vi "Delete Alarm archive and Create Header for new one Alarm archive.vi"(8 "error in":errorcluster) -> (0 "error out":errorcluster)   [LabVIEW 2023]
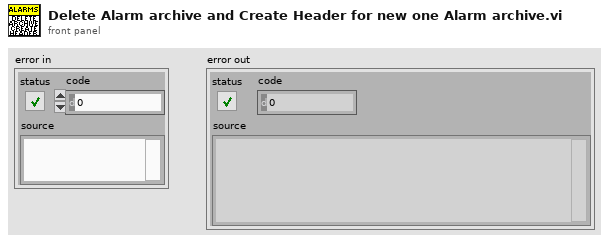
[diagram p1: front panel]
types:
  T1 = enum16{"open", "replace", "create", "open or create", "replace or create", "replace or create with confirmation"}
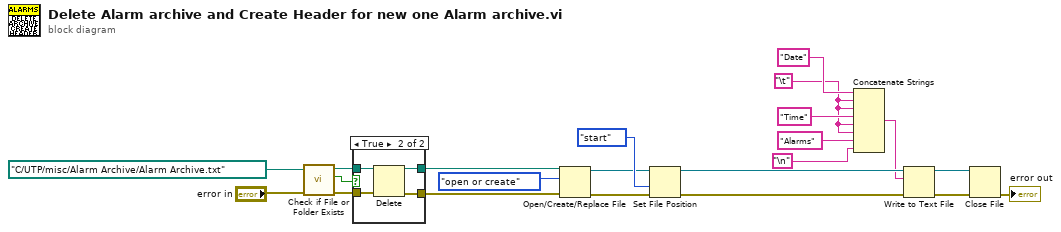
[diagram p0: block diagram]
diagram:
  w12 = "\t"
  n1 = call <vilib>:"Check if File or Folder Exists.vi"("error in (no error)"="error in", "path"=path "C:/UTP/misc/Alarm Archive/Alarm Archive.txt" ("file path (use dialog)")) -> ("error out"=w1:errorcluster, "file or folder exists?"=w2:bool, "dup path"=w3:path)  [unwired: 7 in]
  n2 = case shown="True" w2 {
    tunnel: [w24 w28] -> w7
    tunnel: [w23 w27] -> w6
    tunnel: w3 -> [w24 w26]
    tunnel: w1 -> [w23 w25]
    frame False {
    }
    frame True {
      n3 = Delete(path (use dialog)=w26, error in=w25) -> (deleted path=w28:path, error out=w27:errorcluster)  [unwired: 3 in, 1 out]
    }
  }
  n4 = Open/Create/Replace File(file path (use dialog)=w7, error in=w6, operation (0:open)=T1."open or create") -> (refnum out=w9:refnum<file>, error out=w8:errorcluster)  [unwired: 3 in, 1 out]
  n5 = Set File Position(refnum=w9, from (0:start)=enum16{"start", "end", "current"}."start", error in=w8) -> (refnum out=w20:refnum<file>, error out=w19:errorcluster)  [unwired: 1 in]
  n6 = Concatenate Strings("Date" ("string"), w12, w12, "Time" ("string"), w12, w12, "Alarms" ("string"), "\n") -> (w15:string)
  n7 = Write to Text File(file (use dialog)=w20, text=w15, error in=w19) -> (refnum out=w18:refnum<file>, error out=w17:errorcluster)  [unwired: 1 in, 1 out]
  n8 = Close File(refnum=w18, error in=w17) -> (error out=→"error out":errorcluster)  [unwired: 1 out]
